vi "Update Selected Heads.vi"(8 "error in (no error)":errorcluster, 10 "Selected Heads":string, 11 "Test in":refnum<class "Test.lvclass">) -> (0 "error out":errorcluster, 3 "Test out":refnum<class "Test.lvclass">)   [LabVIEW 2019, in "Test.lvlib" / "Test.lvclass"]
uses:
  Test.lvclass
  Test.lvclass/Test.ctl
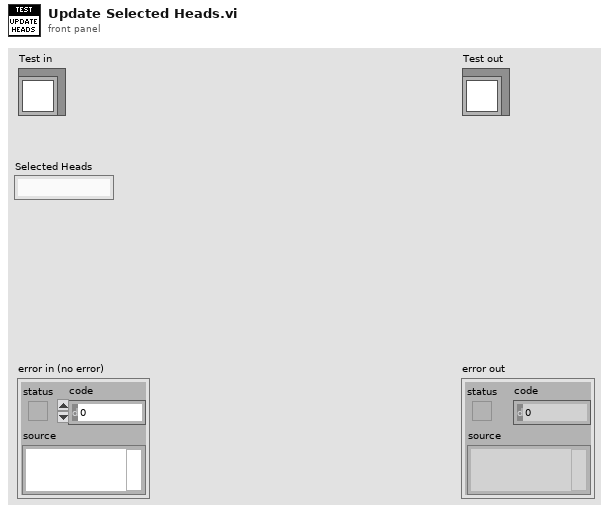
[diagram p1: front panel]
types:
  T1 = map{string, cluster{"Selected Heads":string, "Instrument":refnum<class "Message Enqueuer.lvclass">, "Platform":refnum<class "Message Enqueuer.lvclass">}}
  T2 = cluster{"Selected Heads":string, "Instrument":refnum<class "Message Enqueuer.lvclass">, "Platform":refnum<class "Message Enqueuer.lvclass">}
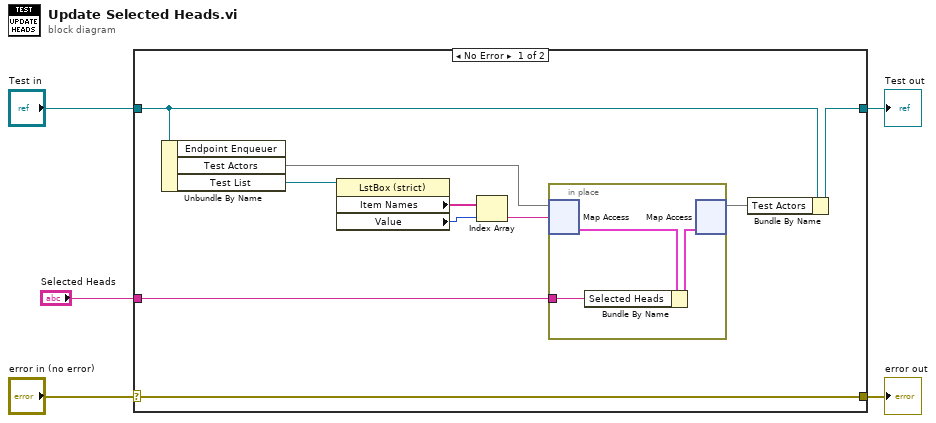
[diagram p0: block diagram]
diagram:
  n1 = case shown="No Error" "error in (no error)" {
    selector: "error in (no error)" -> [w15 w20]
    tunnel: [w15 w20] -> w4
    tunnel: [w8 w19] -> w2
    tunnel: "Test in" -> [w9 w19]
    tunnel: "Selected Heads" -> [w6 _]
    frame No Error {
      n2 = Unbundle By Name(w9) -> ("Test Actors"=w14:T1, "Test List"=w11:refnum<vi>)  [unwired: 1 out]
      n3 = property class="LstBox (strict)"(reference=w11) -> ("Item Names"=w10:string[], "Value"=w12:i32)  [unwired: 1 in, 2 out]
      n4 = Index Array(array=w10, index=w12) -> (element=w13:string)
      n5 = in-place {
        in-place-border: w6 -> [w17]
        n6 = in-place-map #1(w14, w13) -> (w18:T2)  [unwired: 1 in, 1 out]
        n7 = Bundle By Name(cluster=w18, "Selected Heads"=w17) -> (w16:T2)
        n8 = in-place-map #1(w16) -> (w7:T1)  [unwired: 1 in, 2 out]
      }
      n9 = Bundle By Name(cluster=w9, "Test Actors"=w7) -> (w8:refnum<class "Test.lvclass">)
    }
    frame Error {
    }
  }
  "error out" <- w4
  "Test out" <- w2
